vi "Dequeue ECU Action.vi"(8 "error in":errorcluster) -> (0 "error out":errorcluster, 1 "Data":variant, 2 "Message":string)   [LabVIEW 2024, in "RT Management.lvlib"]
uses:
  RT Management.lvlib
  ECU Internal Communications/Queues - Get.vi
  ECU Internal Communications/ECU InterComm.lvlib
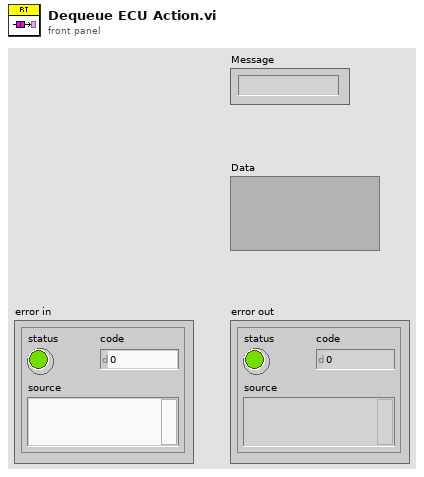
[diagram p1: front panel]
types:
  T1 = typedef "ECU InterComm.lvlib/Process Queues.ctl" = cluster{"Incoming Requests":refnum<queue>, "ECU Working Mode":refnum<queue>}
  T2 = typedef "ECU InterComm.lvlib/QMH Item.ctl" = cluster{"Message":string, "Data":variant}
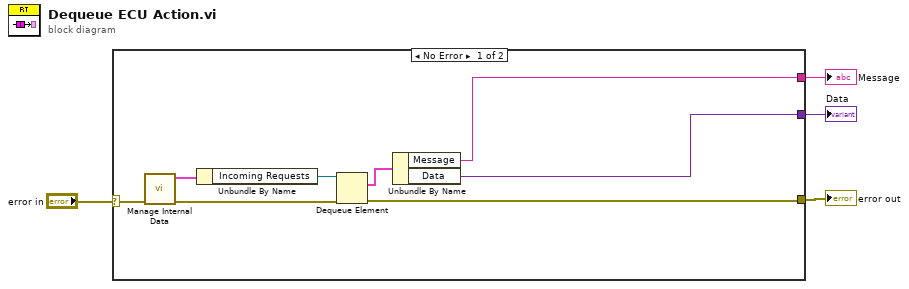
[diagram p0: block diagram]
diagram:
  n1 = case shown="No Error" "error in" {
    selector: "error in" -> [w11 w13]
    tunnel: [w6 w13] -> w3
    tunnel: [w7 _] -> w4
    tunnel: [w5 _] -> w1
    frame No Error {
      n2 = call-poly "Manage Internal Data.vi"("error in"=w11) -> ("error out"=w10:errorcluster, "Queues Out"=w12:T1)  [unwired: 9 in]
      n3 = Unbundle By Name(w12) -> ("Incoming Requests"=w9:refnum<queue>)
      n4 = Dequeue Element(queue=w9, error in (no error)=w10) -> (element=w8:T2, error out=w6:errorcluster)  [unwired: 1 in, 2 out]
      n5 = Unbundle By Name(w8) -> ("Message"=w7:string, "Data"=w5:variant)
    }
    frame Error {
    }
  }
  "error out" <- w3
  "Message" <- w4
  "Data" <- w1
